vi "Get Lidar Data Approx Angle.vi"(9 "Lidar magnitude data":dbl[](array[numeric]), 10 "Lidar angle data":dbl[](array[numeric]), 11 "Desired Angle":dbl) -> (2 "Magnitude":dbl, 3 "Angle":dbl)   [LabVIEW 2016]
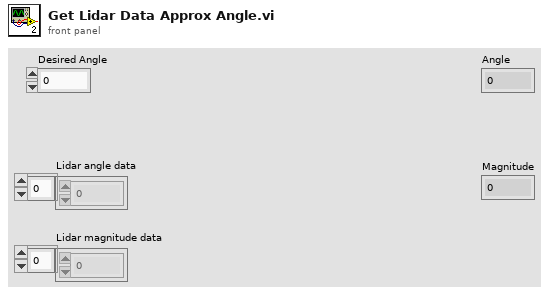
[diagram p1: front panel]
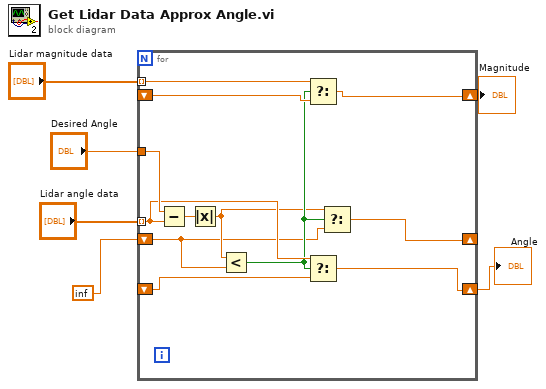
[diagram p0: block diagram]
diagram:
  n1 = for {
    tunnel: "Lidar angle data" -> [w13] mode=indexing
    tunnel: "Desired Angle" -> [w18]
    tunnel: "Lidar magnitude data" -> [w16] mode=indexing
    shift-right: [w12] -> w3
    shift-left: _ -> [w8]
    shift-right: [w15] -> w2
    shift-left: _ -> [w14]
    shift-right: [w9] -> _
    shift-left: inf -> [w7]
    n2 = Subtract(x=w18, y=w13) -> (x-y=w17:dbl)
    n3 = Absolute Value(x=w17) -> (abs(x)=w10:dbl)
    n4 = Less?(x=w10, y=w7) -> (x < y?=w11:bool)
    n5 = Select(t=w16, s=w11, f=w14) -> (s? t:f=w15:dbl)
    n6 = Select(t=w13, s=w11, f=w8) -> (s? t:f=w12:dbl)
    n7 = Select(t=w10, s=w11, f=w7) -> (s? t:f=w9:dbl)
  }
  "Angle" <- w3
  "Magnitude" <- w2
